vi "niFpga_GUIDs.vi"() -> ()   [LabVIEW 2018]
panel:
  in  "GUID_VivadoProjectExportBuildSpec":string="{2B20A4C3-BFB3-48A1-8780-1C27A3A2B812}"
  in  "GUID_Fpga":string="{B824FFC7-1B3E-4521-A49E-679E3411987D}"
  in  "GUID_SimulationBuildSpec":string="{F4C2B394-C5C5-4996-B2AA-F856A474C101}"
  in  "GUID_VI":string="{D60740D6-F254-4BBC-5675-8858F35B810E}"
  in  "GUID_CompilationBuildSpec":string="{F4C5E96F-7410-48A5-BB87-3559BC9B167F}"
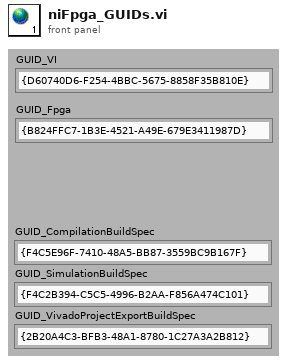
[diagram p1: front panel]
diagram:
